vi "Button Toggle Servo.vi"(11 "Boolean":bool) -> (3 "Camera Angle":i32)   [LabVIEW 2023]
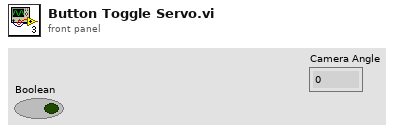
[diagram p1: front panel]
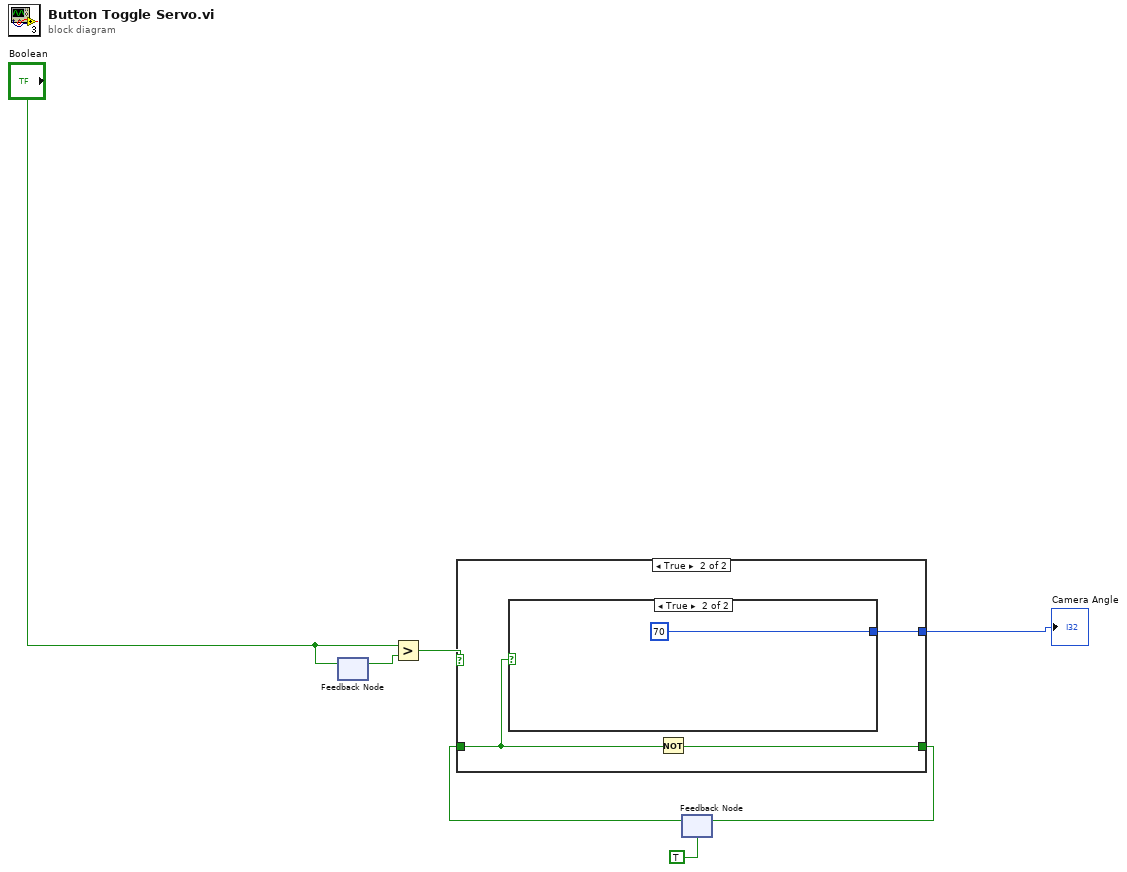
[diagram p0: block diagram]
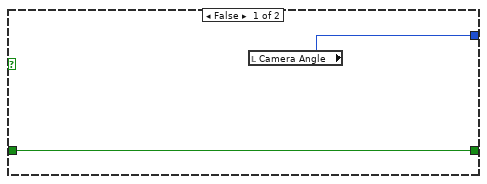
[diagram p2: hidden frame]
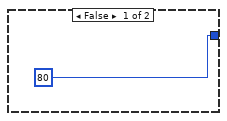
[diagram p3: hidden frame]
diagram:
  n1 = feedback #1() -> (w3:bool)  [unwired: 1 in]
  n2 = feedback-in #1("Boolean") -> ()
  n3 = Greater?(x="Boolean", y=w3) -> (0:w2:bool)
  n4 = feedback #2(TRUE) -> (w4:bool)
  n5 = case shown="True" w2 {
    tunnel: w4 -> [w9 w11]
    tunnel: [w9 w12] -> w5
    tunnel: [w8 w10] -> w1
    frame False {
      n6 = local read "Camera Angle"() -> (w8:i32)
    }
    frame True {
      n7 = case shown="True" w11 {
        tunnel: [80 70] -> w10
        frame False {
        }
        frame True {
        }
      }
      n8 = Not(x=w11) -> (.not. x?=w12:bool)
    }
  }
  "Camera Angle" <- w1
  n9 = feedback-in #2(w5) -> ()
